vi "Module Top Level_jhlee.vi"(8 "error in":errorcluster) -> (0 "error out":errorcluster)   [LabVIEW 2020, in "Error Handler.lvlib"]
doc: "This is the top level of the error handler module (a free running module of the ATM simulator). \n\nIt is closed using a user event or a local Stop button. It communicates with the other modules using a\nqueue based API which has comms modules that can be swapped if required."
uses:
  Error Handler.lvlib
  Private Controls/Module Data Cluster.ctl
  Private Controls/Module Action.ctl
  User Events/Controls/UE Abort Action.ctl
panel:
  in  "Path":path=path "C:/Users/user/Google 드라이브/Jeonghwa/Labview/Labiview 2018/CLA/Sample Exams/ATM (100528-01)/Solution (LV 2013)/Modules/Error Handler/Error log.csv"
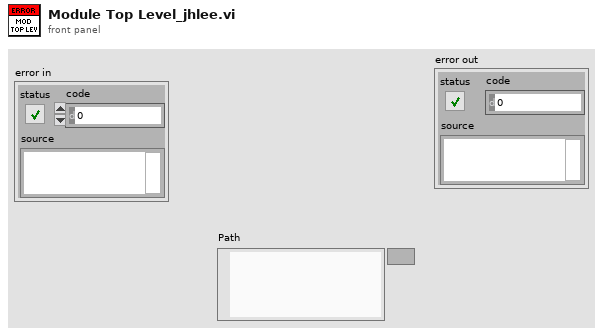
[diagram p1: front panel]
types:
  T1 = typedef "Error Handler.lvlib/Module Data Cluster.ctl" = cluster{"Data":variant, "Action":T2}
  T2 = typedef "Error Handler.lvlib/Module Action.ctl" = enum16{"Process_Step_Err", "Sensor_IO_err", "User_Console_err", "Display_Consol_err", "Error_Log", "Error", "Exit", "Init"}
  T3 = enum16{"open", "replace", "create", "open or create", "replace or create", "replace or create with confirmation"}
  T4 = typedef "UE Abort Action.ctl" = enum16{"Destroy", "Get", "Create"}
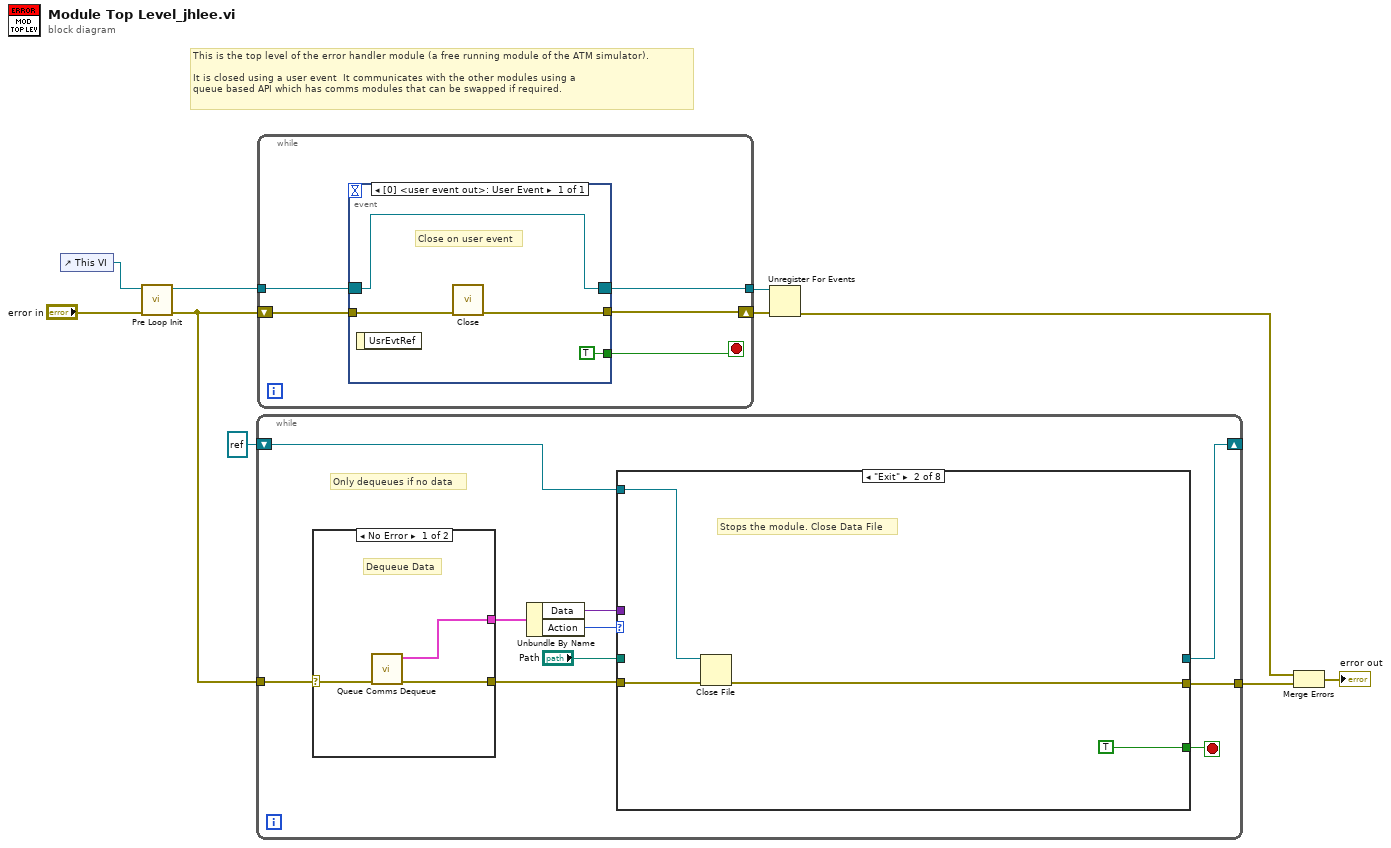
[diagram p0: block diagram]
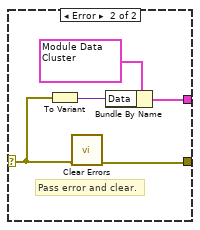
[diagram p2: hidden frame]
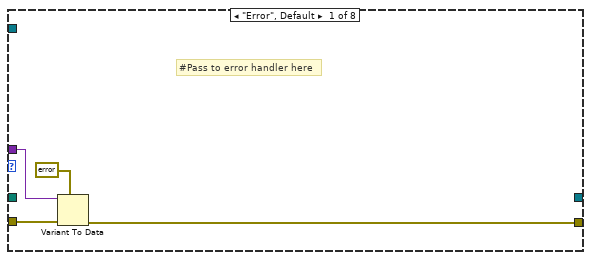
[diagram p3: hidden frame]
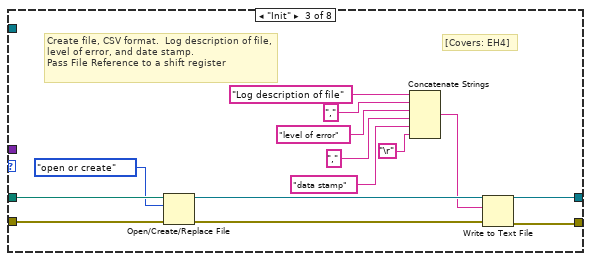
[diagram p4: hidden frame]
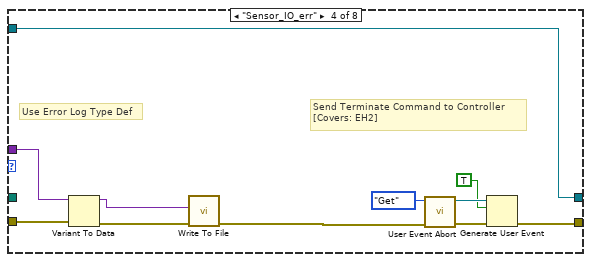
[diagram p5: hidden frame]
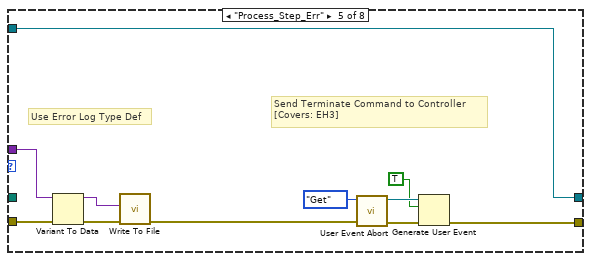
[diagram p6: hidden frame]
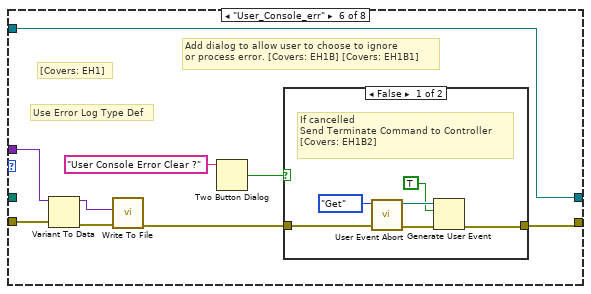
[diagram p7: hidden frame]
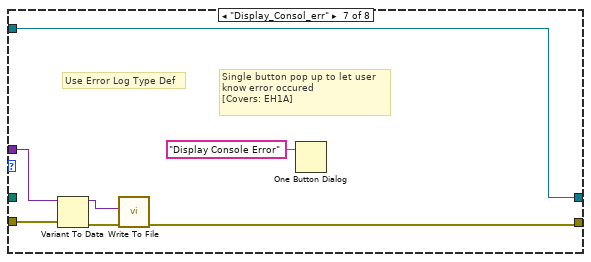
[diagram p9: hidden frame]
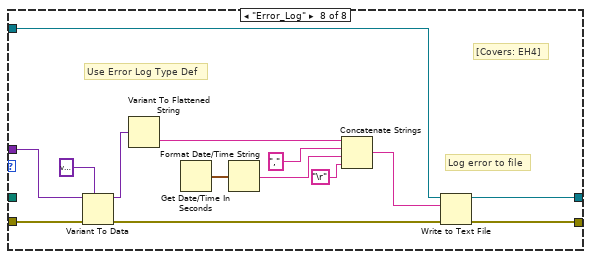
[diagram p10: hidden frame]
diagram:
  # "This is the top level of the error handler module (a free running module of the ATM simulator). \n\nIt is closed using a user event  It communicates with the other modules using a\nqueue based API which has comms modules that can be swapped if required."
  n1 = control-ref of="This VI"() -> (w10:refnum<vi>)
  n2 = call "Pre Loop Init.vi"("error in"="error in", "Ref In"=w10) -> ("error out"=w5:errorcluster, "Event Registration Refnum"=w8:refnum<event-registration>)  [unwired: 8 in]
  n3 = while {
    tunnel: w5 -> [w19]
    tunnel: [w14] -> w3
    shift-right: [w12] -> _
    shift-left: refnum<file> refnum ("refnum out") -> [w11]
    stop <- w20 stop-if-true
    # "Only dequeues if no data"
    n4 = case shown="No Error" w19 {
      selector: w19 -> [w22 w24]
      tunnel: [w23 w25] -> w17
      tunnel: [w21 w26] -> w18
      frame No Error {
        # "Dequeue Data"
        n5 = call "Queue Comms Dequeue.vi"("error in"=w22) -> ("error out"=w23:errorcluster, "Data Out"=w21:T1)  [unwired: 9 in]
      }
      frame Error {
        # "Pass error and clear."
        n6 = To Variant(anything=w24) -> (Variant=w27:variant)
        n7 = call <vilib>:"Clear Errors.vi"("error in (no error)"=w24) -> ("error out"=w25:errorcluster)  [unwired: 5 in, 1 out]
        n8 = Bundle By Name(cluster=T1 {"Data"=variant, "Action"=enum."Error"} ("Cluster"), "Data"=w27) -> (w26:T1)
      }
    }
    n9 = Unbundle By Name(w18) -> ("Data"=w15:variant, "Action"=w16:T2)
    n10 = case shown="\"Exit\"" w16 {
      tunnel: [_ TRUE _ _ _ _ _ _] -> w20
      tunnel: w17 -> [w31 w35 w50 w55 w67 w80 w94 w109]
      tunnel: w15 -> [w32 _ _ w54 w64 w78 w93 w104]
      tunnel: [w30 w34 w38 w56 w63 w73 w89 w98] -> w14
      tunnel: "Path" -> [_ _ w49 _ _ _ _ _]
      tunnel: [_ _ w37 w57 w68 w81 w95 w97] -> w12
      tunnel: w11 -> [_ w33 _ w57 w68 w81 w95 w99]
      frame "Error", Default {
        # "#Pass to error handler here"
        n11 = Variant To Data(error in=w31, type=errorcluster {"status"=FALSE, "code"=0, "source"=""} ("error out"), Variant=w32) -> (error out=w30:errorcluster)  [unwired: 1 out]
      }
      frame "Exit" {
        # "Stops the module. Close Data File"
        n12 = Close File(refnum=w33, error in=w35) -> (error out=w34:errorcluster)  [unwired: 1 out]
      }
      frame "Init" {
        # "[Covers: EH4]"
        # "Create file, CSV format.  Log description of file, level of error, and date stamp.\nPass File Reference to a shift register"
        n13 = Open/Create/Replace File(file path (use dialog)=w49, error in=w50, operation (0:open)=T3."open or create") -> (refnum out=w46:refnum<file>, error out=w47:errorcluster)  [unwired: 3 in, 1 out]
        n14 = Concatenate Strings("Log description of file", ",", "level of error", ",", "data stamp", "\r") -> (w39:string)
        n15 = Write to Text File(file (use dialog)=w46, text=w39, error in=w47) -> (refnum out=w37:refnum<file>, error out=w38:errorcluster)  [unwired: 1 in, 1 out]
      }
      frame "Sensor_IO_err" {
        # "Use Error Log Type Def"
        # "Send Terminate Command to Controller\n[Covers: EH2]"
        n16 = Variant To Data(error in=w55, Variant=w54) -> (data=w53:variant, error out=w52:errorcluster)  [unwired: 1 in]
        n17 = call "Write To File.vi"("error in"=w52, "Data"=w53) -> ("error out"=w51:errorcluster)  [unwired: 9 in]
        n18 = call "User Event Abort.vi"("error in"=w51, "Action"=UE_Abort_Action."Get") -> ("error out"=w60:errorcluster, "user event out"=w59:refnum<user-event>)  [unwired: 8 in]
        n19 = Generate User Event(user event=w59, event data cluster=TRUE ("event data"), error in=w60) -> (error out=w56:errorcluster)  [unwired: 1 in, 1 out]
      }
      frame "Process_Step_Err" {
        # "Use Error Log Type Def"
        # "Send Terminate Command to Controller\n[Covers: EH3]"
        n20 = Variant To Data(error in=w67, Variant=w64) -> (data=w65:variant, error out=w66:errorcluster)  [unwired: 1 in]
        n21 = call "Write To File.vi"("error in"=w66, "Data"=w65) -> ("error out"=w62:errorcluster)  [unwired: 9 in]
        n22 = call "User Event Abort.vi"("error in"=w62, "Action"=UE_Abort_Action."Get") -> ("error out"=w71:errorcluster, "user event out"=w70:refnum<user-event>)  [unwired: 8 in]
        n23 = Generate User Event(user event=w70, event data cluster=TRUE ("event data"), error in=w71) -> (error out=w63:errorcluster)  [unwired: 1 in, 1 out]
      }
      frame "User_Console_err" {
        # "[Covers: EH1]"
        # "Add dialog to allow user to choose to ignore\nor process error. [Covers: EH1B] [Covers: EH1B1]"
        # "Use Error Log Type Def"
        n24 = Variant To Data(error in=w80, Variant=w78) -> (data=w77:variant, error out=w79:errorcluster)  [unwired: 1 in]
        n25 = call "Write To File.vi"("error in"=w79, "Data"=w77) -> ("error out"=w74:errorcluster)  [unwired: 9 in]
        n26 = Two Button Dialog(message="User Console Error Clear ?") -> (T button?=w76:bool)  [unwired: 2 in]
        n27 = case shown="False" w76 {
          tunnel: w74 -> [w83 w88]
          tunnel: [w82 w88] -> w73
          frame False {
            # "If cancelled\nSend Terminate Command to Controller\n[Covers: EH1B2]"
            n28 = call "User Event Abort.vi"("error in"=w83, "Action"=UE_Abort_Action."Get") -> ("error out"=w87:errorcluster, "user event out"=w86:refnum<user-event>)  [unwired: 8 in]
            n29 = Generate User Event(user event=w86, event data cluster=TRUE ("event data"), error in=w87) -> (error out=w82:errorcluster)  [unwired: 1 in, 1 out]
          }
          frame True {
            # "If not cancelled, clear error and continue."
          }
        }
      }
      frame "Display_Consol_err" {
        # "Single button pop up to let user\nknow error occured\n[Covers: EH1A]"
        # "Use Error Log Type Def"
        n30 = Variant To Data(error in=w94, Variant=w93) -> (data=w91:variant, error out=w92:errorcluster)  [unwired: 1 in]
        n31 = call "Write To File.vi"("error in"=w92, "Data"=w91) -> ("error out"=w89:errorcluster)  [unwired: 9 in]
        n32 = One Button Dialog(message="Display Console Error") -> ()  [unwired: 1 in, 1 out]
      }
      frame "Error_Log" {
        # "Log error to file"
        # "Use Error Log Type Def"
        # "[Covers: EH4]"
        n33 = Variant To Data(error in=w109, type=variant, Variant=w104) -> (data=w102:variant, error out=w103:errorcluster)
        n34 = Variant To Flattened String(Variant=w102) -> (data string=w101:string)  [unwired: 1 out]
        n35 = Get Date/Time In Seconds() -> (seconds since 1Jan1904=w108:timestamp)
        n36 = Format Date/Time String(seconds (now)=w108) -> (date/time string=w105:string)  [unwired: 2 in]
        n37 = Concatenate Strings(w101, ",", w105, "\r") -> (w100:string)
        n38 = Write to Text File(file (use dialog)=w99, text=w100, error in=w103) -> (refnum out=w97:refnum<file>, error out=w98:errorcluster)  [unwired: 1 in, 1 out]
      }
    }
  }
  n39 = while {
    shift-right: [w113] -> w7
    shift-left: w5 -> [w114]
    tunnel: w8 -> [w112]
    tunnel: [w111] -> w6
    stop <- w110 stop-if-true
    n40 = event shown="[0] <user event out>: User Event" {
      selector: w112 -> [w118]
      dyn-events: [w118] -> w111
      timeout: _ -> [_]
      tunnel: w114 -> [w117]
      tunnel: [w116] -> w113
      tunnel: [TRUE ("stop")] -> w110
      event User Event {
        # "Close on user event"
        n41 = event-data() -> ()  [unwired: 1 in, 1 out]
        n42 = call "Close.vi"("error in"=w117) -> ("error out"=w116:errorcluster)  [unwired: 10 in]
      }
    }
  }
  n43 = Unregister For Events(event registration refnum=w6, error in=w7) -> (error out=w2:errorcluster)
  n44 = Merge Errors(w2, w3) -> (→"error out":errorcluster)
